vi "Test Agilent U2000.vi"() -> ()   [LabVIEW 2020, in "U2000.lvclass"]
uses:
  U2000.lvclass
  <instrlib>/Agilent U2000 Series/Agilent U2000 Series.lvlib
panel:
  in  "Frequency (5E+7 Hz)":dbl=50000000.0
  out "error out 2":errorcluster
  out "Instrument Driver Revision":string
  out "Instrument Firmware Revision":string
  out "Temperature":dbl
  out "Measurement":dbl
  out "error out":errorcluster
  in  "VISA resource name":refnum<visa-resource-name>
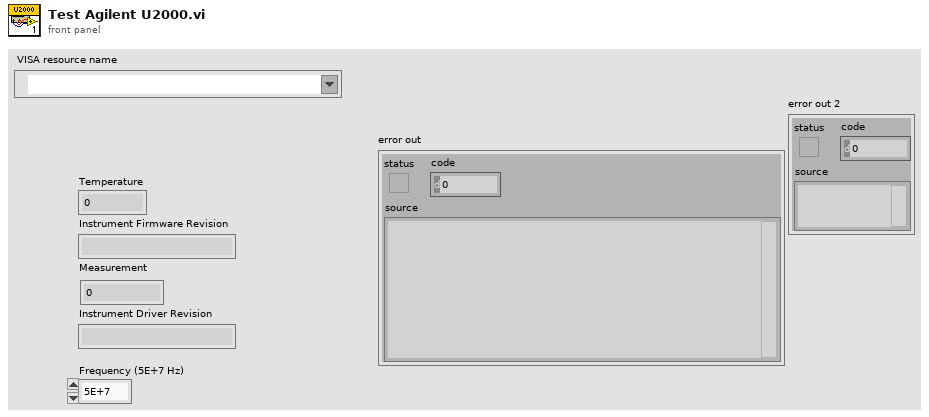
[diagram p1: front panel]
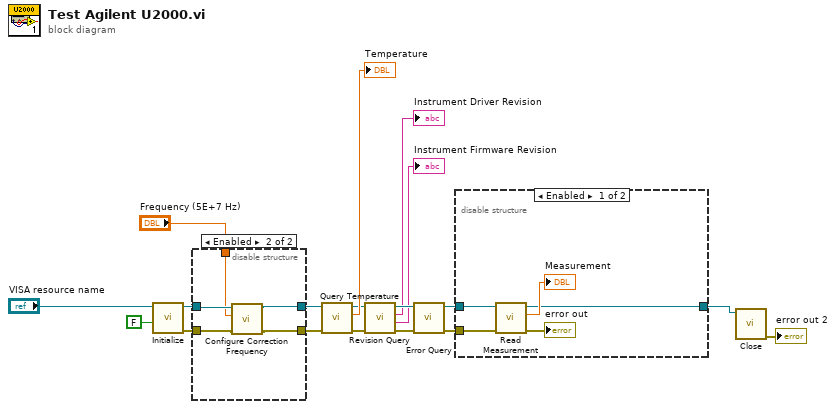
[diagram p0: block diagram]
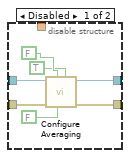
[diagram p2: hidden frame]
diagram:
  n1 = call <instrlib>:"Initialize.vi"("Reset (True)"=FALSE, "VISA resource name"="VISA resource name") -> ("error out"=w6:errorcluster, "VISA resource name out"=w7:refnum<visa-resource-name>)  [unwired: 8 in]
  n2 = disable-structure shown="Enabled" {
    disable-tunnel: w7 -> [w25 w29]
    disable-tunnel: w6 -> [w24 w30]
    disable-tunnel: [w23 w28] -> w5
    disable-tunnel: [w22 w27] -> w4
    disable-tunnel: "Frequency (5E+7 Hz)" -> [_ w26]
    frame Disabled {
      n3 = call <instrlib>:"Configure Averaging.vi"("Enable Step Detection (T: Enable)"=TRUE, "Auto Averaging (T: Enable)"=FALSE, "Enable Averaging (T: Enable)"=FALSE, "error in (no error)"=w24, "VISA resource name"=w25) -> ("error out"=w22:errorcluster, "VISA resource name out"=w23:refnum<visa-resource-name>)  [unwired: 5 in]
    }
    frame Enabled {
      n4 = call <instrlib>:"Configure Correction Frequency.vi"("error in (no error)"=w30, "Frequency (5E+7 Hz)"=w26, "VISA resource name"=w29) -> ("error out"=w27:errorcluster, "VISA resource name out"=w28:refnum<visa-resource-name>)  [unwired: 7 in]
    }
  }
  n5 = call <instrlib>:"Query Temperature.vi"("error in (no error)"=w4, "VISA resource name"=w5) -> ("error out"=w12:errorcluster, "Temperature"=→"Temperature":dbl, "VISA resource name out"=w13:refnum<visa-resource-name>)  [unwired: 7 in]
  n6 = call <instrlib>:"Revision Query.vi"("error in (no error)"=w12, "VISA resource name"=w13) -> ("error out"=w10:errorcluster, "Instrument Firmware Revision"=→"Instrument Firmware Revision":string, "Instrument Driver Revision"=→"Instrument Driver Revision":string, "VISA resource name out"=w11:refnum<visa-resource-name>)  [unwired: 6 in]
  n7 = call <instrlib>:"Error Query.vi"("error in (no error)"=w10, "VISA resource name"=w11) -> ("error out"=w14:errorcluster, "VISA resource name out"=w15:refnum<visa-resource-name>)  [unwired: 6 in, 2 out]
  n8 = disable-structure shown="Enabled" {
    disable-tunnel: w14 -> [w33 _]
    disable-tunnel: w15 -> [w32 w36]
    disable-tunnel: [w31 w36] -> w3
    frame Enabled {
      n9 = call <instrlib>:"Read Measurement.vi"("error in (no error)"=w33, "VISA resource name"=w32) -> ("error out"=→"error out":errorcluster, "Measurement"=→"Measurement":dbl, "VISA resource name out"=w31:refnum<visa-resource-name>)  [unwired: 7 in]
    }
    frame Disabled {
    }
  }
  n10 = call <instrlib>:"Close.vi"("VISA resource name"=w3) -> ("error out"=→"error out 2":errorcluster)  [unwired: 10 in]
